vi "Get_Vi_Data.vi"(4 "bypass":bool, 6 "error in (no error) 2":errorcluster, 7 "port number":u16=3374, 8 "Data Type":u16(ring) items=["String", "Double", "Boolean", "Variant"], 9 "VI name":string, 10 "Control Name":string, 11 "Data mac ip address":string) -> (0 "error out":errorcluster, 1 "Boolean":bool, 2 "Data (Double)":dbl format="%#_4g", 3 "Data (String)":string, 5 "Data (Variant)":variant)   [LabVIEW 2025]
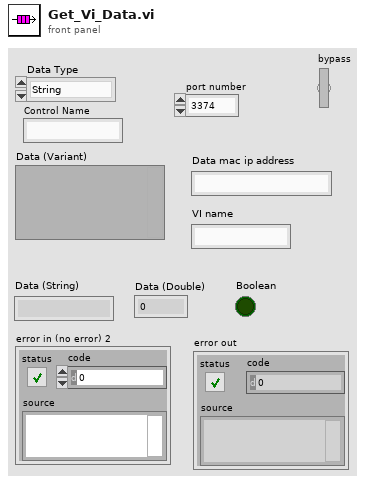
[diagram p1: front panel]
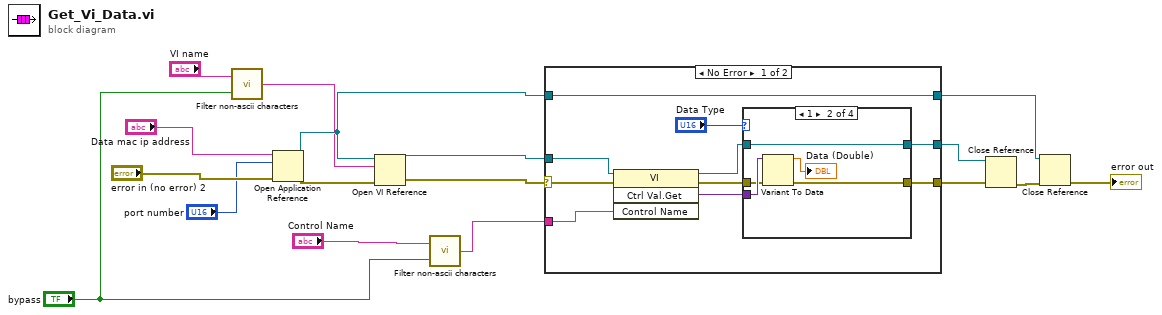
[diagram p0: block diagram]
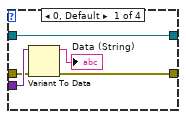
[diagram p2: hidden frame]
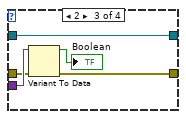
[diagram p3: hidden frame]
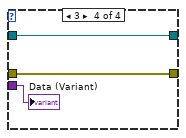
[diagram p4: hidden frame]
diagram:
  n1 = call "Filter non-ascii characters.vi"("bypass"="bypass", 2:"VI name") -> ("output"=w3:string)
  n2 = Open Application Reference(8:"error in (no error) 2", 10:"port number", 11:"Data mac ip address") -> (0:w12:errorcluster, 3:w15:refnum<vi>)  [unwired: 1 in]
  n3 = Open VI Reference(application reference (local)=w15, vi path=w3, error in (no error)=w12) -> (vi reference=w17:refnum<vi>, error out=w16:errorcluster)  [unwired: 3 in]
  n4 = call "Filter non-ascii characters.vi"("bypass"="bypass", 2:"Control Name") -> ("output"=w5:string)
  n5 = case shown="No Error" w16 {
    selector: w16 -> [w22 w47]
    tunnel: w17 -> [w27 w48]
    tunnel: [w21 w47] -> w14
    tunnel: [w20 w48] -> w8
    tunnel: [w19 w46] -> w7
    tunnel: w15 -> [w19 w46]
    tunnel: w5 -> [w18 _]
    frame No Error {
      n6 = invoke class="VI" method="Ctrl Val.Get"(reference=w27, error in=w22, "Control Name"=w18) -> (reference out=w23:refnum<vi>, error out=w24:errorcluster, "Get Control Value Variant"=w25:variant)  [unwired: 1 in, 1 out]
      n7 = case shown="1" "Data Type" {
        tunnel: w25 -> [w32 w37 w42 w45]
        tunnel: w24 -> [w31 w36 w41 w44]
        tunnel: w23 -> [w28 w33 w38 w43]
        tunnel: [w29 w34 w39 w44] -> w21
        tunnel: [w28 w33 w38 w43] -> w20
        frame 0, Default {
          n8 = Variant To Data(error in=w31, Variant=w32) -> (data=→"Data (String)":string, error out=w29:errorcluster)  [unwired: 1 in]
        }
        frame 1 {
          n9 = Variant To Data(error in=w36, Variant=w37) -> (data=→"Data (Double)":dbl, error out=w34:errorcluster)  [unwired: 1 in]
        }
        frame 2 {
          n10 = Variant To Data(error in=w41, Variant=w42) -> (data=→"Boolean":bool, error out=w39:errorcluster)  [unwired: 1 in]
        }
        frame 3 {
          "Data (Variant)" <- w45
        }
      }
    }
    frame Error {
    }
  }
  n11 = Close Reference(reference=w8, error in (no error)=w14) -> (error out=w13:errorcluster)
  n12 = Close Reference(reference=w7, error in (no error)=w13) -> (error out=→"error out":errorcluster)
